vi "Write Log Line.vi"(10 "log line":string, 11 "file handler in":refnum<class "File Handler.lvclass">) -> (0 "error out":errorcluster, 3 "file handler out":refnum<class "File Handler.lvclass">)   [LabVIEW 2024, in "Logging.lvlib" / "File Handler.lvclass"]
uses:
  File Handler.lvclass
  File Handler.lvclass/File Handler.ctl
panel:
  # "Connector Pane"
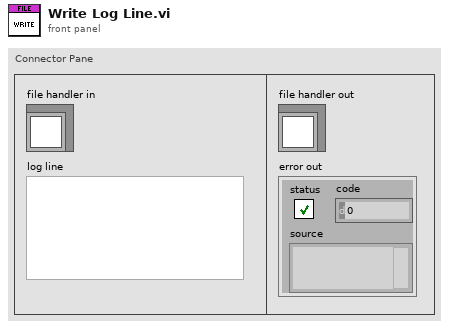
[diagram p1: front panel]
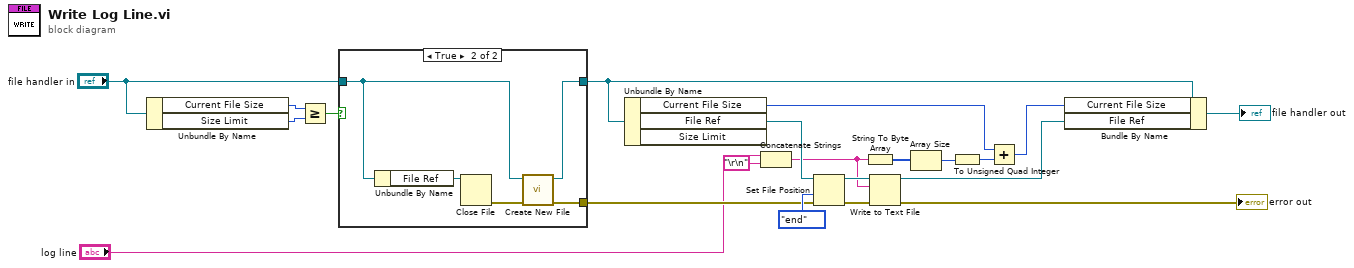
[diagram p0: block diagram]
diagram:
  n1 = Unbundle By Name("file handler in") -> ("Current File Size"=w9:u64, "Size Limit"=w8:u64)
  n2 = Greater Or Equal?(x=w9, y=w8) -> (x >= y?=w5:bool)
  n3 = case shown="True" w5 {
    tunnel: "file handler in" -> [w22 w24]
    tunnel: [_ w27] -> w7
    tunnel: [w22 w26] -> w6
    frame False {
    }
    frame True {
      n4 = Unbundle By Name(w24) -> ("File Ref"=w23:refnum<file>)
      n5 = Close File(refnum=w23) -> (error out=w25:errorcluster)  [unwired: 1 in, 1 out]
      n6 = call "Create New File.vi"("error in (no error)"=w25, "file handler in"=w24) -> ("error out"=w27:errorcluster, "file handler out"=w26:refnum<class "File Handler.lvclass">)  [unwired: 8 in]
    }
  }
  n7 = Unbundle By Name(w6) -> ("Current File Size"=w13:u64, "File Ref"=w17:refnum<file>)  [unwired: 1 out]
  n8 = Concatenate Strings("log line", "\r\n") -> (w11:string)
  n9 = Set File Position(refnum=w17, from (0:start)=enum16{"start", "end", "current"}."end", error in=w7) -> (refnum out=w20:refnum<file>, error out=w21:errorcluster)  [unwired: 1 in]
  n10 = String To Byte Array(string=w11) -> (unsigned byte array=w16:u8[])
  n11 = Write to Text File(file (use dialog)=w20, text=w11, error in=w21) -> (refnum out=w18:refnum<file>, error out=→"error out":errorcluster)  [unwired: 1 in, 1 out]
  n12 = Array Size(array=w16) -> (size(s)=w15:i32)
  n13 = To Unsigned Quad Integer(1:w15) -> (0:w14:u64)
  n14 = Add(x=w13, y=w14) -> (x+y=w10:u64)
  n15 = Bundle By Name(cluster=w6, "Current File Size"=w10, "File Ref"=w18) -> (→"file handler out":refnum<class "File Handler.lvclass">)
